vi "Reset.vi"(8 "error in (no error)":errorcluster, 11 "VISA resource name":refnum<visa-resource-name>) -> (0 "error out":errorcluster, 3 "VISA resource name out":refnum<visa-resource-name>)   [LabVIEW 2011, in "Tektronix 7000 Series.lvlib"]
doc: "Resets the instrument. This VI then waits 1200 ms for the reset operation to complete and then sends a set of default setup commands to the instrument. If your oscilloscope can not finish the operation within 1200ms, you can increase the time."
uses:
  Tektronix 7000 Series.lvlib
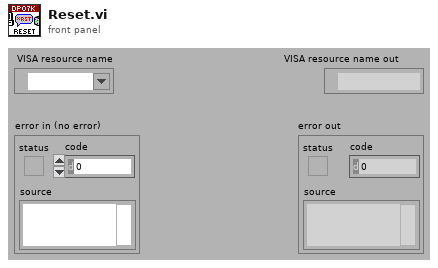
[diagram p1: front panel]
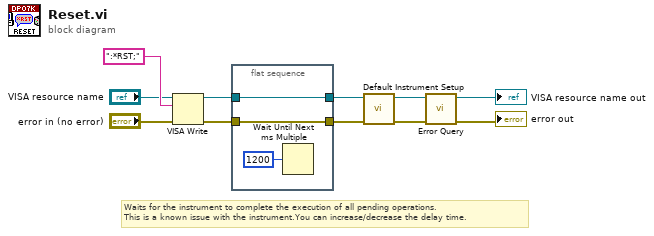
[diagram p0: block diagram]
diagram:
  # "Waits for the instrument to complete the execution of all pending operations.\nThis is a known issue with the instrument.You can increase/decrease the delay time."
  n1 = VISA Write(VISA resource name="VISA resource name", write buffer=":*RST;", error in (no error)="error in (no error)") -> (VISA resource name out=w4:refnum<visa-resource-name>, error out=w3:errorcluster)  [unwired: 1 out]
  n2 = flat-sequence {
    tunnel: w4 -> [w13]
    tunnel: [w13] -> w2
    tunnel: w3 -> [w12]
    tunnel: [w12] -> w1
    frame #0 {
      n3 = Wait Until Next ms Multiple(millisecond multiple=u32 1200) -> ()  [unwired: 1 out]
    }
  }
  n4 = call "Default Instrument Setup.vi"("error in (no error)"=w1, "VISA resource name"=w2) -> ("error out"=w7:errorcluster, "VISA resource name out"=w8:refnum<visa-resource-name>)  [unwired: 8 in]
  n5 = call "Error Query.vi"("error in (no error)"=w7, "VISA resource name"=w8) -> ("error out"=→"error out":errorcluster, "VISA resource name out"=→"VISA resource name out":refnum<visa-resource-name>)  [unwired: 6 in, 2 out]
